vi "transform_rotation.vi"(4 "Transform":T1) -> (1 "Rotation":T1=[[1.0, 0.0, 0.0], [0.0, 1.0, 0.0], [0.0, 0.0, 1.0]])   [LabVIEW 2013]
uses:
  <vilib>/Analysis/Matrix/Datatypes/RealMatrix.ctl
  <vilib>/Analysis/Matrix/NI_Matrix.lvlib
panel:
  # "Extract rotation part of a transform matrix."
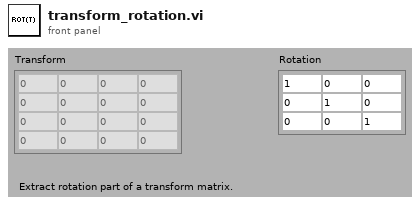
[diagram p1: front panel]
types:
  T1 = typedef "NI_Matrix.lvlib/RealMatrix.ctl" = dbl[][]
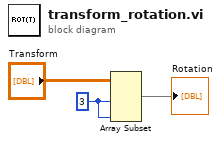
[diagram p0: block diagram]
diagram:
  w1 = 3 ("index")
  n1 = Array Subset(array="Transform", length (row)=w1, length (col)=w1) -> (→"Rotation":T1)  [unwired: 2 in]
